vi "Sub Sequence A.vi"(7 "Socket":i32, 8 "error in (no error)":errorcluster) -> (0 "error out":errorcluster)   [LabVIEW 2019, in "Multisocket Example(Station2).lvlib"]
uses:
  Multisocket Example(Station2).lvlib
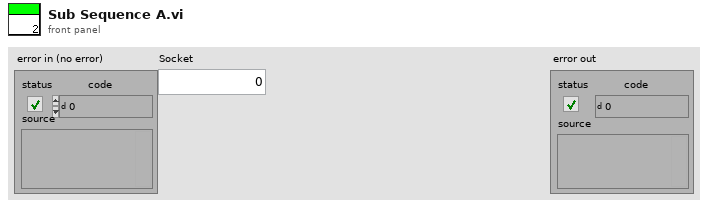
[diagram p1: front panel]
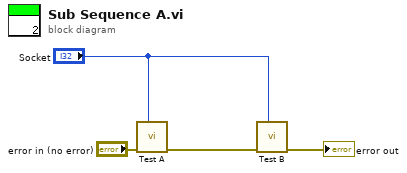
[diagram p0: block diagram]
diagram:
  n1 = call "Test A.vi"("Socket"="Socket", "error in (no error)"="error in (no error)") -> ("error out"=w3:errorcluster)  [unwired: 9 in]
  n2 = call "Test B.vi"("Socket"="Socket", "error in (no error)"=w3) -> ("error out"=→"error out":errorcluster)  [unwired: 9 in]
